vi "Add Folder to Targets.vi"(7 "Folder Name":string="NI VeriStand APIs", 8 "error in (no error)":errorcluster, 9 "Content Paths":path[](array[path]), 10 "Target Names":string[](array[string]), 11 "Project Sync Tools in":refnum<class "Project Sync Tools.lvclass">) -> (0 "error out":errorcluster, 3 "Project Sync Tools out":refnum<class "Project Sync Tools.lvclass">)   [LabVIEW 2019, in "Project Sync Tools.lvclass"]
uses:
  Project Sync Tools.lvclass
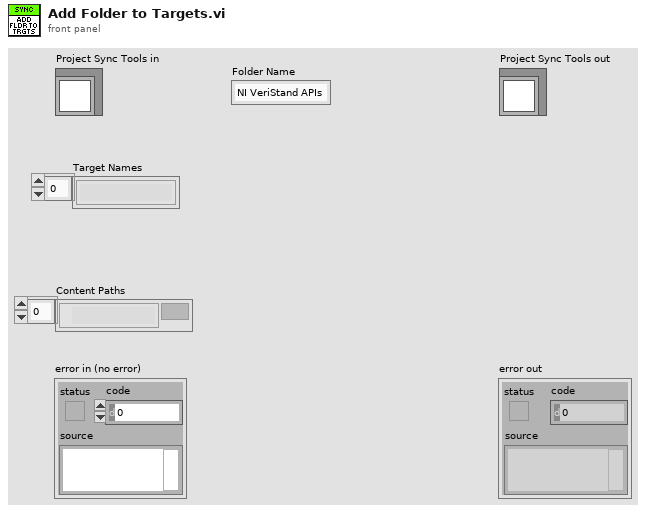
[diagram p1: front panel]
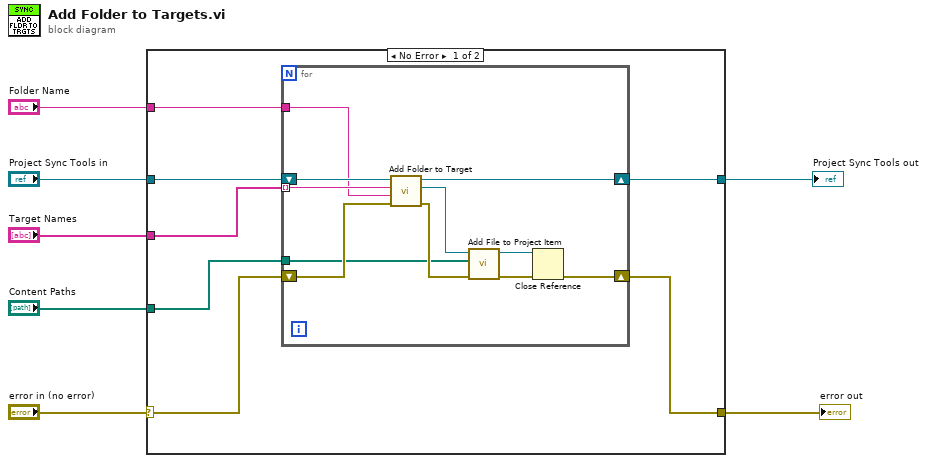
[diagram p0: block diagram]
diagram:
  n1 = case shown="No Error" "error in (no error)" {
    selector: "error in (no error)" -> [w9 w27]
    tunnel: [w8 w27] -> w6
    tunnel: [w12 w26] -> w4
    tunnel: "Project Sync Tools in" -> [w13 w26]
    tunnel: "Folder Name" -> [w14 _]
    tunnel: "Target Names" -> [w11 _]
    tunnel: "Content Paths" -> [w10 _]
    frame No Error {
      n2 = for {
        tunnel: w11 -> [w23] mode=indexing
        shift-right: [w22] -> w12
        shift-left: w13 -> [w24]
        shift-right: [w16] -> w8
        shift-left: w9 -> [w25]
        tunnel: w10 -> [w19]
        tunnel: w14 -> [w15]
        n3 = call "Add Folder to Target.vi"("error in (no error)"=w25, "Name"=w15, "Target Name"=w23, "Project Sync Tools in"=w24) -> ("error out"=w21:errorcluster, "Folder Item ref"=w20:refnum<vi>, "Project Sync Tools out"=w22:refnum<class "Project Sync Tools.lvclass">)  [unwired: 5 in]
        n4 = call "Add File to Project Item.vi"("error in"=w21, "File Paths"=w19, "Item ref in"=w20) -> ("error out"=w18:errorcluster, "Item ref out"=w17:refnum<vi>)  [unwired: 7 in]
        n5 = Close Reference(reference=w17, error in (no error)=w18) -> (error out=w16:errorcluster)
      }
    }
    frame Error {
    }
  }
  "error out" <- w6
  "Project Sync Tools out" <- w4
